vi "Write Dictionary Elements (Loop).vi"(8 "error in (no error)":errorcluster, 10 "Data in":T1[](array[typedef]), 11 "Control Experiment in":refnum<class "Control Experiment.lvclass">) -> (0 "error out":errorcluster, 3 "Control Experiment out":refnum<class "Control Experiment.lvclass">)   [LabVIEW 2019, in "Control Experiment.lvclass"]
uses:
  Control Experiment.lvclass
  <userlib>/LevyLab/LV-Data/LV-Data/Typedefs/Dictionary--cluster.ctl
  <userlib>/LevyLab/LV-Data/LV-Data/LV-Data.lvclass
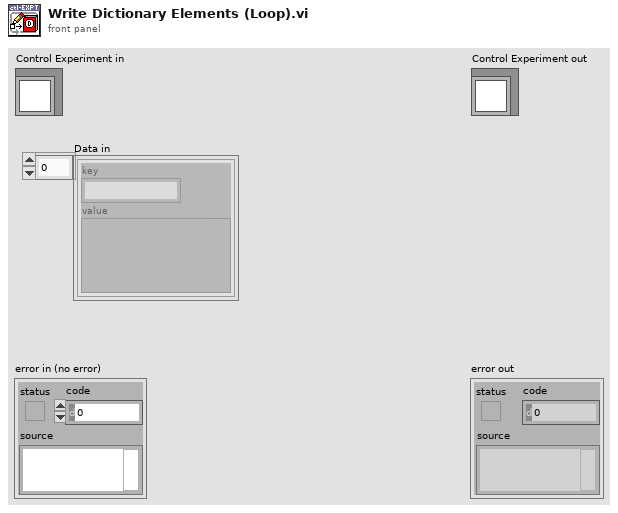
[diagram p1: front panel]
types:
  T1 = typedef "LV-Data.lvclass/Dictionary--cluster.ctl" = cluster{"key":string, "value":variant}
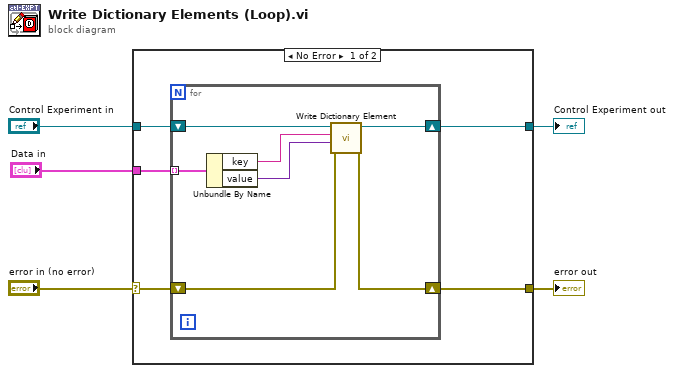
[diagram p0: block diagram]
diagram:
  n1 = case shown="No Error" "error in (no error)" {
    selector: "error in (no error)" -> [w8 w18]
    tunnel: [w7 w18] -> w4
    tunnel: [w9 w19] -> w2
    tunnel: "Control Experiment in" -> [w10 w19]
    tunnel: "Data in" -> [w6 _]
    frame No Error {
      n2 = for {
        shift-right: [w16] -> w9
        shift-left: w10 -> [w17]
        shift-right: [w14] -> w7
        shift-left: w8 -> [w15]
        tunnel: w6 -> [w13] mode=indexing
        n3 = Unbundle By Name(w13) -> ("key"=w12:string, "value"=w11:variant)
        n4 = call "Write Dictionary Element.vi"("error in (no error)"=w15, "value"=w11, "key"=w12, "Control Experiment in"=w17) -> ("error out"=w14:errorcluster, "Control Experiment out"=w16:refnum<class "Control Experiment.lvclass">)  [unwired: 6 in]
      }
    }
    frame Error {
    }
  }
  "error out" <- w4
  "Control Experiment out" <- w2
